vi "Register.vi"(10 "element (unused)":T1, 11 "data in":refnum<class "EventMessengerPData.lvclass">) -> (2 "Event Registration Refnum":refnum<event-registration>, 3 "data out":refnum<class "EventMessengerPData.lvclass">)   [LabVIEW 2020, in "Event Messenger Priority.lvlib" / "EventMessengerPData.lvclass"]
uses:
  EventMessengerPData.lvclass
  EventMessengerPData.lvclass/EventMessengerPData.ctl
  Event Data.ctl
  Event Messenger Priority.lvlib
  Element.ctl
panel:
  # "See note on block diagram."
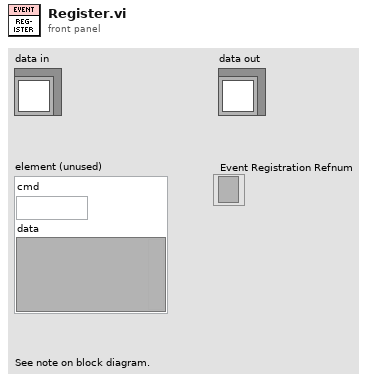
[diagram p1: front panel]
types:
  T1 = typedef "Event Messenger Priority.lvlib/Element.ctl" = cluster{"cmd":string, "data":variant}
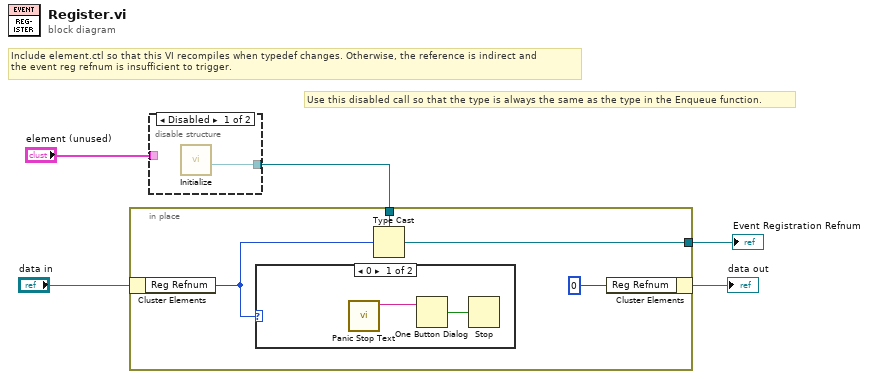
[diagram p0: block diagram]
diagram:
  # "Include element.ctl so that this VI recompiles when typedef changes. Otherwise, the reference is indirect and\nthe event reg refnum is insufficient to trigger."
  # "Use this disabled call so that the type is always the same as the type in the Enqueue function."
  n1 = disable-structure shown="Disabled" {
    disable-tunnel: [w6 _] -> w2
    disable-tunnel: "element (unused)" -> [_ _]
    frame Disabled {
      n2 = call "Initialize.vi"() -> ("Event Registration Refnum"=w6:refnum<event-registration>)  [unwired: 10 in, 1 out]
    }
    frame Enabled {
    }
  }
  n3 = in-place {
    in-place-border: [w8] -> w3
    in-place-border: w2 -> [w7]
    n4 = in-place-cluster #1("data in") -> ("Reg Refnum"=w9:u32)
    n5 = case shown="0" w9 {
      frame 0 {
        n6 = call "Panic Stop Text.vi"() -> ("Text"=w11:string)  [unwired: 11 in]
        n7 = One Button Dialog(message=w11) -> (true=w12:bool)  [unwired: 1 in]
        n8 = Stop(stop? (T)=w12) -> ()
      }
      frame Default {
      }
    }
    n9 = Type Cast(type=w7, x=w9) -> (*(type *) &x=w8:refnum<event-registration>)
    n10 = in-place-cluster #1("Reg Refnum"=u32 0) -> (→"data out":refnum<class "EventMessengerPData.lvclass">)
  }
  "Event Registration Refnum" <- w3
